vi "main TEST PURPOSES ONLY.vi"() -> ()   [LabVIEW 2013, in "Client Controller.lvlib" / "Client Controller.lvclass"]
uses:
  Client Controller.lvclass
  <vilib>/ActorFramework/Message Queue/Message Queue.lvclass/Message Queue.ctl
  <vilib>/ActorFramework/Message Enqueuer/Message Enqueuer.lvclass/Message Enqueuer.ctl
  <vilib>/ActorFramework/Message Enqueuer/Enqueue.vi
  <vilib>/ActorFramework/Message Priority Queue/Priority Enqueue.vi
  <vilib>/ActorFramework/Message Enqueuer/Message Enqueuer.lvclass
  <vilib>/ActorFramework/Stop Msg/Stop Msg.lvclass
  <vilib>/ActorFramework/Message Queue/Message Queue.lvclass
  <vilib>/ActorFramework/Actor/Actor.lvclass
panel:
  in  "Number of Clients":i32=5
  in  "Stop All":bool
  out "error out":errorcluster
  # "This version of 'main.vi' is intended for use to test\nconnectivity of large numbers of simultaneous clients. \nIt makes it easy to stop them all simultaneously."
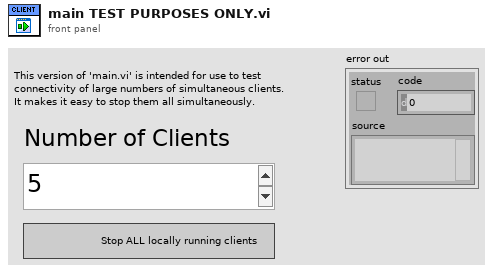
[diagram p1: front panel]
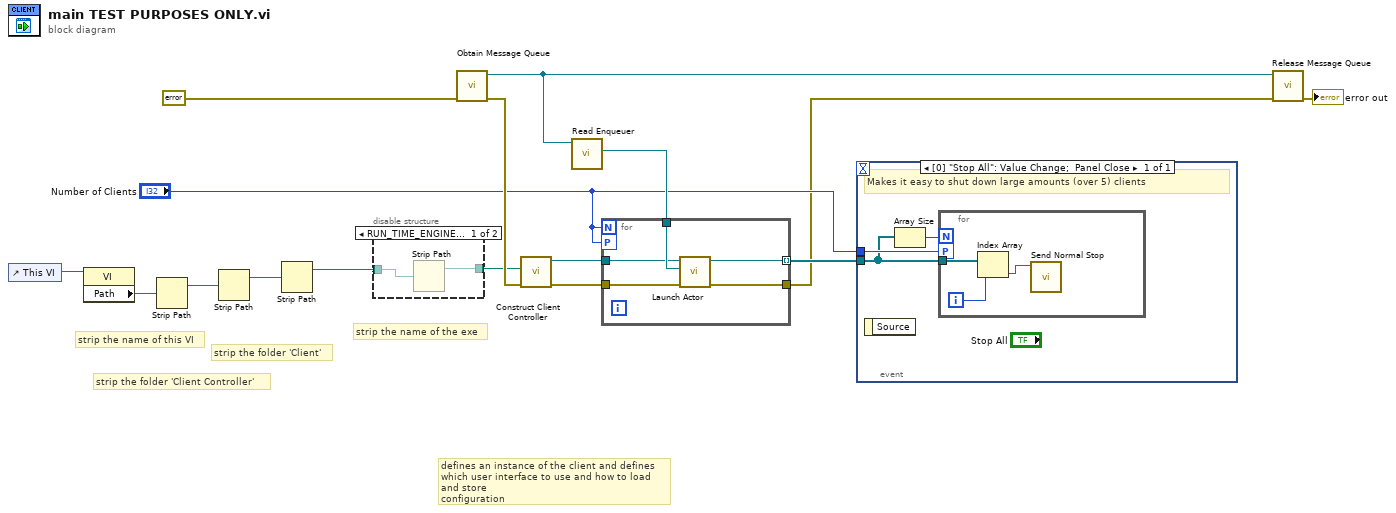
[diagram p0: block diagram]
diagram:
  # "strip the name of the exe"
  # "defines an instance of the client and defines which user interface to use and how to load and store\nconfiguration"
  # "strip the folder 'Client'"
  # "strip the folder 'Client Controller'"
  # "strip the name of this VI"
  n1 = control-ref of="This VI"() -> (w11:refnum<vi>)
  n2 = property class="VI"(reference=w11) -> ("Path"=w16:path)  [unwired: 1 in, 2 out]
  n3 = Strip Path(path=w16) -> (stripped path=w15:path)  [unwired: 1 out]
  n4 = Strip Path(path=w15) -> (stripped path=w14:path)  [unwired: 1 out]
  n5 = Strip Path(path=w14) -> (stripped path=w13:path)  [unwired: 1 out]
  n6 = disable-structure "Conditional Disable Structure" shown="RUN_TIME_ENGINE==True" {
    disable-tunnel: w13 -> [w18 w19]
    disable-tunnel: [w17 w19] -> w4
    frame condition #0 {
      n7 = Strip Path(path=w18) -> (stripped path=w17:path)  [unwired: 1 out]
    }
    frame condition #1 (active) {
    }
  }
  n8 = call <vilib>:"Obtain Message Queue.vi"("error in (no error)"=errorcluster {"status"=FALSE, "code"=0, "source"=""}) -> ("error out"=w6:errorcluster, "Message Queue"=w10:refnum<class "Message Queue.lvclass">)  [unwired: 9 in]
  n9 = call "Construct Client Controller.vi"("error in (no error)"=w6, "Base Path"=w4) -> ("error out"=w2:errorcluster, "Client Controller out"=w5:refnum<class "Client Controller.lvclass">)  [unwired: 8 in]
  n10 = call <vilib>:"Read Enqueuer.vi"("Message Queue"=w10) -> ("Message Enqueuer"=w8:refnum<class "Message Enqueuer.lvclass">)  [unwired: 10 in]
  n11 = for {
    N: "Number of Clients" -> [_]
    tunnel: w8 -> [w24]
    tunnel: w5 -> [w23]
    tunnel: [w22] -> w7 mode=indexing
    workers-P: "Number of Clients" -> [_]
    tunnel: w2 -> [w21]
    tunnel: [w20] -> w1
    n12 = call <vilib>:"Launch Actor.vi"("error in (no error)"=w21, "Actor-to-Caller Enqueuer"=w24, "Actor"=w23) -> ("error out"=w20:errorcluster, "Caller-To-Actor Enqueuer"=w22:refnum<class "Message Enqueuer.lvclass">)  [unwired: 7 in]
  }
  n13 = event shown="[0] \"Stop All\": Value Change;  Panel Close" {
    selector: _ -> [_]
    dyn-events: _ -> [_]
    timeout: _ -> [_]
    tunnel: w7 -> [w25]
    tunnel: "Number of Clients" -> [w27]
    event "Stop All": Value Change; Panel Close {
      # "Makes it easy to shut down large amounts (over 5) clients"
      n14 = event-data() -> ()  [unwired: 1 in, 1 out]
      n15 = Array Size(array=w25) -> (size(s)=w26:i32)
      n16 = for {
        N: w26 -> [_]
        tunnel: w25 -> [w29]
        workers-P: w27 -> [_]
        i -> [w30]
        n17 = Index Array(array=w29, index=w30) -> (element=w28:refnum<class "Message Enqueuer.lvclass">)
        n18 = call <vilib>:"Send Normal Stop.vi"("Message Enqueuer"=w28) -> ()  [unwired: 10 in, 1 out]
      }
    }
  }
  n19 = call <vilib>:"Release Message Queue.vi"("error in (no error)"=w1, "Message Queue"=w10) -> ("error out"=→"error out":errorcluster)  [unwired: 8 in, 1 out]
